vi "Configure Digital Input Noise Bandwidth.vi"(8 "error in (no error)":errorcluster, 9 "Carrier Bandwidth (1.00000000E+0 Hz)":dbl=1.0 format="%.8e", 10 "Flat Noise Bandwidth (1.00000000E+0 Hz)":dbl=1.0 format="%.8e", 11 "VISA resource name":refnum<visa-resource-name>) -> (0 "error out":errorcluster, 3 "VISA resource name out":refnum<visa-resource-name>)   [LabVIEW 2018, in "Agilent PSG MXG Series.lvlib"]
doc: "Configures the flat noise bandwidth of the real-time noise for an ARB waveform and the carrier bandwidth over which the additive white gaussian noise (AWGN) is applied.\n\n<b>Note:</b>\nIt is applicable for N5172B/82B with <b>Option 004</b> only."
uses:
  Agilent PSG MXG Series.lvlib
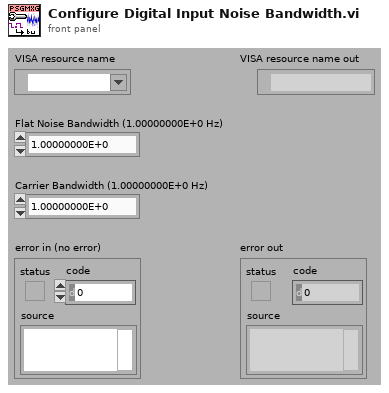
[diagram p1: front panel]
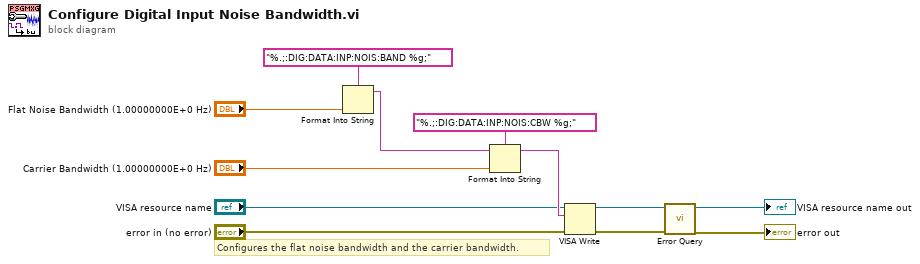
[diagram p0: block diagram]
diagram:
  # "Configures the flat noise bandwidth and the carrier bandwidth."
  n1 = Format Into String(format string="%.;:DIG:DATA:INP:NOIS:BAND %g;", "Flat Noise Bandwidth (1.00000000E+0 Hz)") -> (resulting string=w10:string)  [unwired: 2 in, 1 out]
  n2 = Format Into String(format string="%.;:DIG:DATA:INP:NOIS:CBW %g;", initial string=w10, "Carrier Bandwidth (1.00000000E+0 Hz)") -> (resulting string=w7:string)  [unwired: 1 in, 1 out]
  n3 = VISA Write(VISA resource name="VISA resource name", write buffer=w7, error in (no error)="error in (no error)") -> (VISA resource name out=w4:refnum<visa-resource-name>, error out=w3:errorcluster)  [unwired: 1 out]
  n4 = call "Error Query.vi"("error in (no error)"=w3, "VISA resource name"=w4) -> ("error out"=→"error out":errorcluster, "VISA resource name out"=→"VISA resource name out":refnum<visa-resource-name>)  [unwired: 6 in, 2 out]
